vi "Save Recall Spurious Emission Parameter.vi"(0 "VISA resource name":refnum<visa-resource-name>, 5 "Spurious Emission Operation (0:Save)":i32(ring) items=["Save", "Recall"], 7 "Register (1)":i32=1 min=1 max=8, 11 "error in (no error)":errorcluster) -> (4 "VISA resource name out":refnum<visa-resource-name>, 15 "error out":errorcluster)   [LabVIEW 2020, in "Anritsu Signal Analyzer Series.lvlib"]
doc: "Saves or recalls the Spurious Emission Parameter"
uses:
  Anritsu Signal Analyzer Series.lvlib
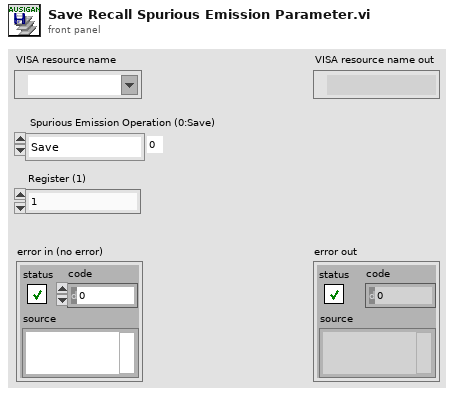
[diagram p1: front panel]
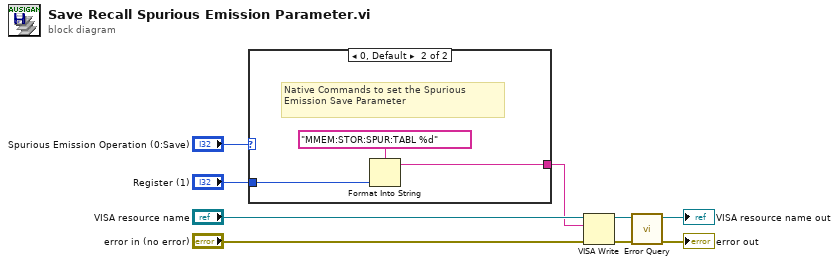
[diagram p0: block diagram]
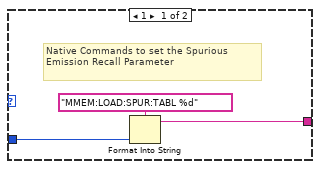
[diagram p2: hidden frame]
diagram:
  n1 = case shown="0, Default" "Spurious Emission Operation (0:Save)" {
    tunnel: "Register (1)" -> [w12 w15]
    tunnel: [w10 w14] -> w2
    frame 1 {
      # "Native Commands to set the Spurious Emission Recall Parameter"
      n2 = Format Into String(format string="MMEM:LOAD:SPUR:TABL %d" ("_CommandSet"), w12) -> (resulting string=w10:string)  [unwired: 2 in, 1 out]
    }
    frame 0, Default {
      # "Native Commands to set the Spurious Emission Save Parameter"
      n3 = Format Into String(format string="MMEM:STOR:SPUR:TABL %d" ("_CommandSet"), w15) -> (resulting string=w14:string)  [unwired: 2 in, 1 out]
    }
  }
  n4 = VISA Write(VISA resource name="VISA resource name", write buffer=w2, error in (no error)="error in (no error)") -> (VISA resource name out=w3:refnum<visa-resource-name>, error out=w4:errorcluster)  [unwired: 1 out]
  n5 = call "Error Query.vi"("error in (no error)"=w4, "VISA resource name"=w3) -> ("error out"=→"error out":errorcluster, "VISA resource name out"=→"VISA resource name out":refnum<visa-resource-name>)  [unwired: 6 in, 2 out]
